vi "calculate zoom to roi.vi"(11 "Coordinates":i32[](array[numeric])) -> (3 "output cluster":T1)   [LabVIEW 2017]
doc: "SciScan 1.2 160622"
uses:
  Custom Controls/pixel resolution enum.ctl
  GFG/GFGnumericGet.vi
  GFG/GFG library.lvlib
panel:
  out "y.pixel.sz":dbl
  out "x.pixel.sz":dbl
  out "y pixels":dbl
  out "y offset":dbl
  out "x offset":dbl
  out "voltage top":dbl
  out "voltage bottom":dbl
  out "voltage right":dbl
  out "voltage left":dbl
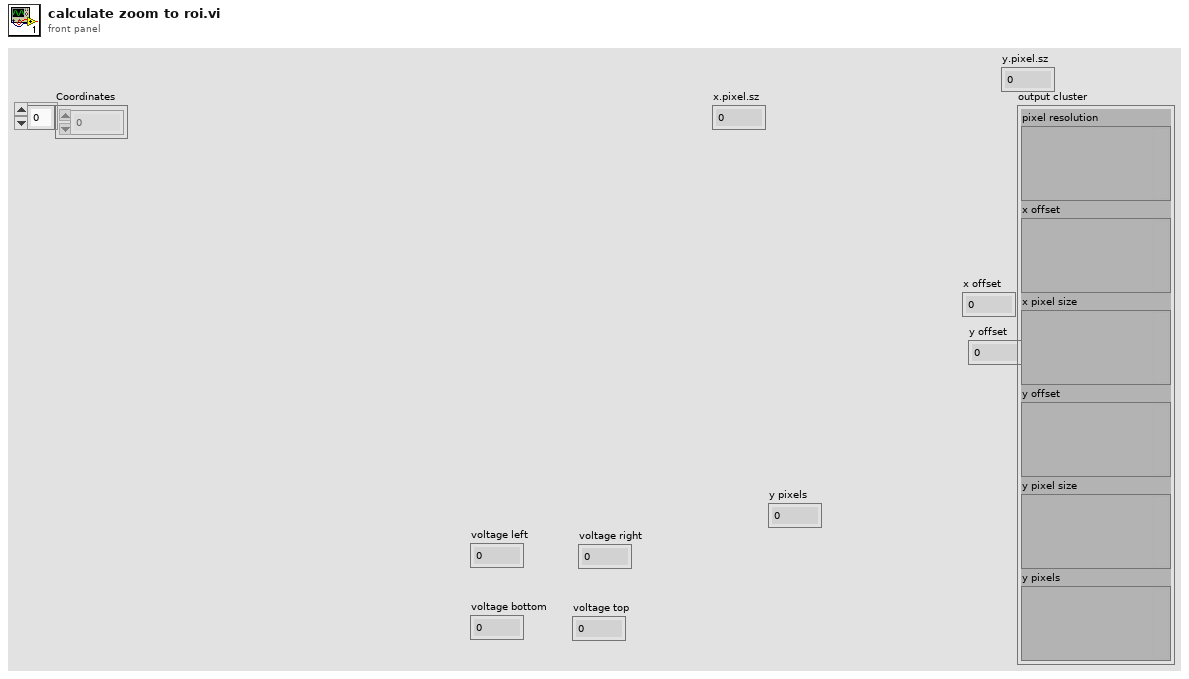
[diagram p1: front panel]
types:
  T1 = cluster{"pixel resolution":variant, "x offset":variant, "x pixel size":variant, "y offset":variant, "y pixel size":variant, "y pixels":variant}
  T2 = typedef "pixel resolution enum.ctl" = enum16{"128 x 128", "256 x 128", "256 x 256", "512 x  64", "512 x 128", "512 x 256", "512 x 512", "1024 x 512", "1024 x 1024", "arbitrary"}
  T3 = cluster{"xyvoltagefor2frames":dbl[][][], "x.pixels":dbl, "nomin.x.pixels":dbl, "y.pixels":dbl, "fill.fraction":dbl, "x.bidirectional":bool, "y.bidirectional":bool}
  T4 = cluster{"Variant":variant, "Variant":variant, "Variant":variant, "Variant":variant, "Variant":variant, "Variant":variant}
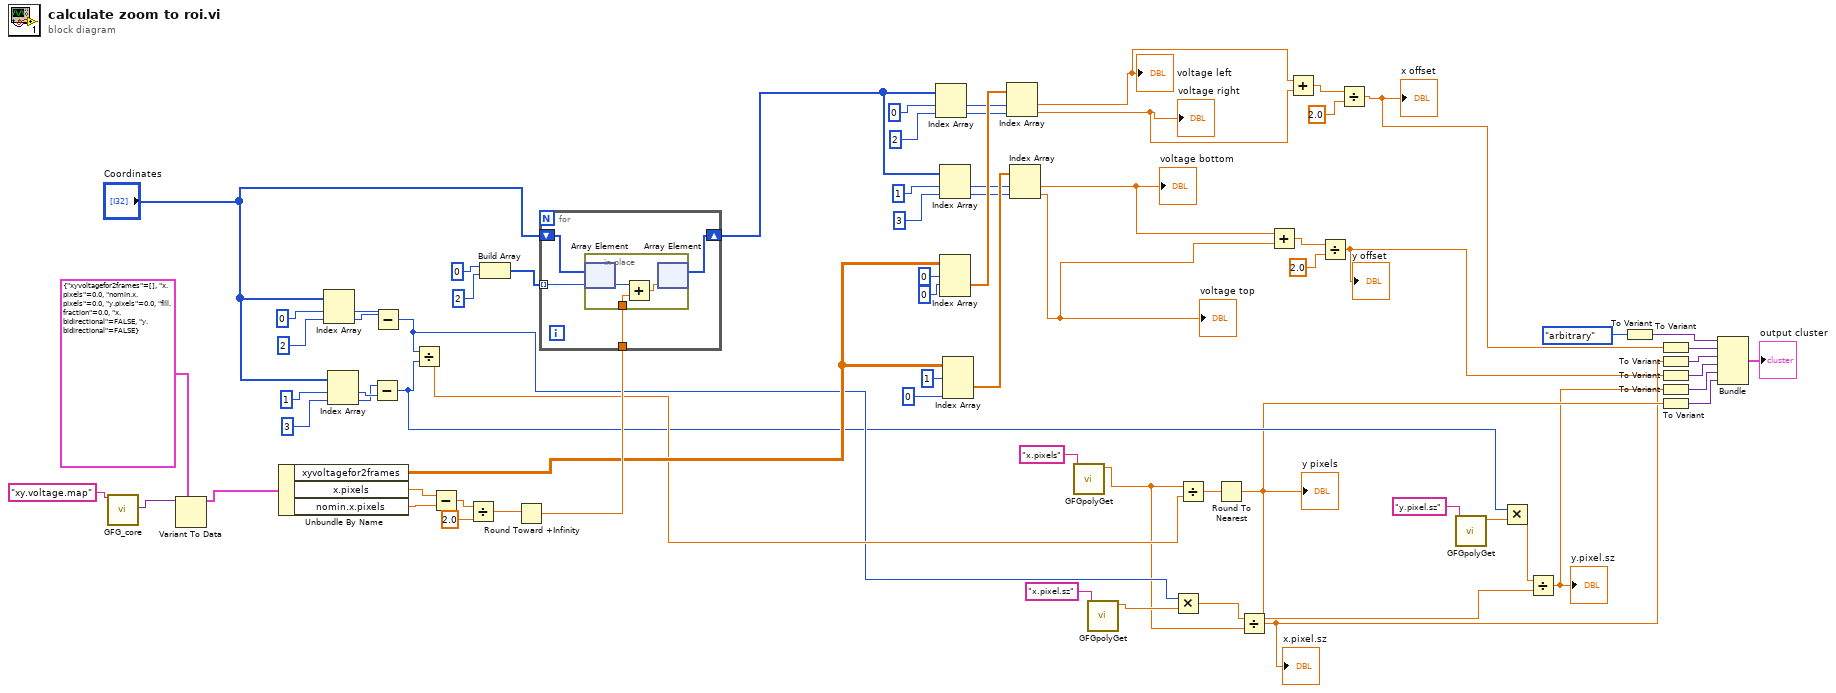
[diagram p0: block diagram]
diagram:
  n1 = call "GFG_core.vi"("Variable Name in"="xy.voltage.map") -> ("Variant Out"=w70:variant)  [unwired: 12 in, 6 out]
  n2 = Variant To Data(type=T3 {"xyvoltagefor2frames"=[], "x.pixels"=0.0, "nomin.x.pixels"=0.0, "y.pixels"=0.0, "fill.fraction"=0.0, "x.bidirectional"=FALSE, "y.bidirectional"=FALSE} ("output cluster"), Variant=w70) -> (data=w68:T3)  [unwired: 1 in, 1 out]
  n3 = Unbundle By Name(w68) -> ("xyvoltagefor2frames"=w55:dbl[][][], "x.pixels"=w66:dbl, "nomin.x.pixels"=w67:dbl)
  n4 = Index Array(array="Coordinates", index #1=0, index #2=2) -> (element #1=w30:i32, element #2=w29:i32)
  n5 = Index Array(array="Coordinates", index #1=1, index #2=3) -> (element #1=w28:i32, element #2=w27:i32)
  n6 = Subtract(x=w27, y=w28) -> (x-y=w4:i32)
  n7 = Subtract(x=w29, y=w30) -> (x-y=w11:i32)
  n8 = Divide(x=w11, y=w4) -> (x/y=w25:dbl)
  n9 = Subtract(x=w66, y=w67) -> (x-y=w65:dbl)
  n10 = Divide(x=w65, y=2.0) -> (x/y=w63:dbl)
  n11 = Build Array(0, 2) -> (w59:i32[])
  n12 = Round Toward +Infinity(x=w63) -> (ceil(x): smallest int >= x=w62:dbl)
  n13 = for {
    tunnel: w62 -> [w75]
    shift-right: [w73] -> w49
    shift-left: "Coordinates" -> [w74]
    tunnel: w59 -> [w72] mode=indexing
    n14 = in-place {
      in-place-border: w75 -> [w77]
      n15 = in-place-array #1(w74, w72) -> (w78:i32)
      n16 = Add(x=w78, y=w77) -> (x+y=w76:dbl)
      n17 = in-place-array #1(w76) -> (w73:i32[])  [unwired: 1 out]
    }
  }
  n18 = Index Array(array=w49, index #1=0, index #2=2) -> (element #1=w47:i32, element #2=w46:i32)
  n19 = Index Array(array=w49, index #1=1, index #2=3) -> (element #1=w44:i32, element #2=w43:i32)
  n20 = Index Array(array=w55, index (dim 0)=0 ("index (page)"), index (dim 1)=0 ("disabled index (row)")) -> (element=w48:dbl[])  [unwired: 1 in]
  n21 = Index Array(array=w55, index (dim 0)=1 ("index (page)"), index (dim 2)=0 ("disabled index (row)")) -> (element=w45:dbl[])  [unwired: 1 in]
  n22 = Index Array(array=w48, index #1=w47, index #2=w46) -> (element #1=w35:dbl, element #2=w42:dbl)
  "voltage left" <- w35
  "voltage right" <- w42
  n23 = Index Array(array=w45, index #1=w44, index #2=w43) -> (element #1=w37:dbl, element #2=w36:dbl)
  "voltage bottom" <- w37
  "voltage top" <- w36
  n24 = call-poly "GFGpolyGet.vi"("Variable Name in"="x.pixels") -> ("Numeric"=w8:dbl)  [unwired: 8 in, 2 out]
  n25 = call-poly "GFGpolyGet.vi"("Variable Name in"="x.pixel.sz") -> ("Numeric"=w10:dbl)  [unwired: 8 in, 2 out]
  n26 = Multiply(x=w11, y=w10) -> (x*y=w9:dbl)
  n27 = Divide(x=w8, y=w25) -> (x/y=w24:dbl)
  n28 = Round To Nearest(number=w24) -> (nearest integer value=w3:dbl)
  "y pixels" <- w3
  n29 = Divide(x=w9, y=w8) -> (x/y=w2:dbl)
  "x.pixel.sz" <- w2
  n30 = Add(x=w37, y=w36) -> (x+y=w38:dbl)
  n31 = Add(x=w35, y=w42) -> (x+y=w41:dbl)
  n32 = Divide(x=w38, y=2.0) -> (x/y=w20:dbl)
  "y offset" <- w20
  n33 = Divide(x=w41, y=2.0) -> (x/y=w21:dbl)
  "x offset" <- w21
  n34 = call-poly "GFGpolyGet.vi"("Variable Name in"="y.pixel.sz") -> ("Numeric"=w6:dbl)  [unwired: 8 in, 2 out]
  n35 = Multiply(x=w4, y=w6) -> (x*y=w7:dbl)
  n36 = Divide(x=w7, y=w3) -> (x/y=w1:dbl)
  "y.pixel.sz" <- w1
  n37 = To Variant(anything=pixel_resolution_enum."arbitrary" ("pixel resolution")) -> (Variant=w19:variant)
  n38 = To Variant(anything=w21) -> (Variant=w18:variant)
  n39 = To Variant(anything=w2) -> (Variant=w17:variant)
  n40 = To Variant(anything=w20) -> (Variant=w16:variant)
  n41 = To Variant(anything=w1) -> (Variant=w15:variant)
  n42 = To Variant(anything=w3) -> (Variant=w14:variant)
  n43 = Bundle("Variant"=w19, "Variant"=w18, "Variant"=w17, "Variant"=w16, "Variant"=w15, "Variant"=w14) -> (→"output cluster":T4)  [unwired: 1 in]
